vi "data_averaging.vi"(10 "Reset?":bool, 11 "New data":dbl[](array[numeric])) -> (3 "Output (averaged)":dbl[](array[numeric]))   [LabVIEW 2019]
uses:
  <vilib>/Analysis/baseanly.llb/Mean (DBL).vi
  Global Plantita Parameters.vi
  <vilib>/Analysis/NI_AALBase.lvlib
panel:
  out "Stored":dbl[](array[numeric])
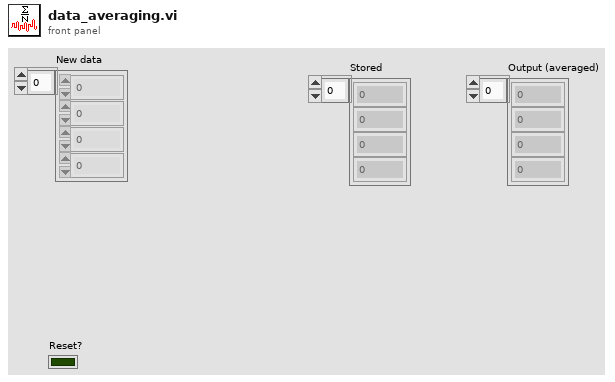
[diagram p1: front panel]
types:
  T1 = cluster{"height_ff (m)":dbl, "C_coag_stock (g/L)":dbl, "flocculation_time(min)":dbl, "clarification_time(min)":dbl, "data_interval (min)":dbl, "kpf":dbl, "kc":dbl, "q":dbl}
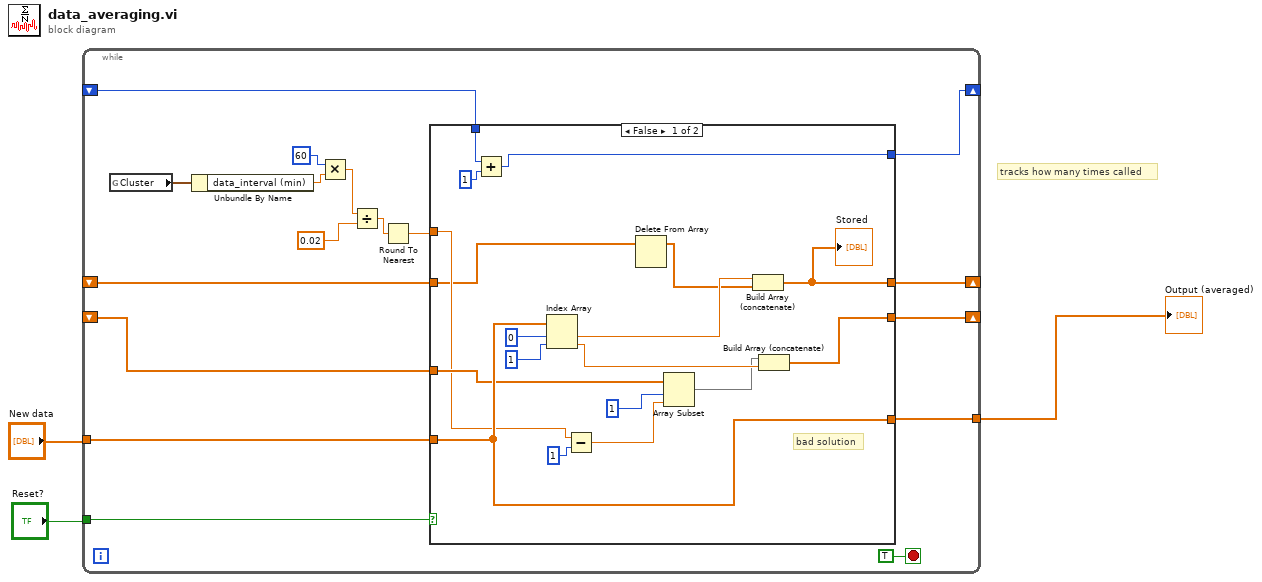
[diagram p0: block diagram]
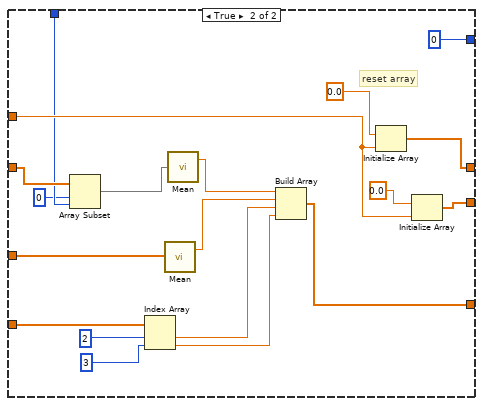
[diagram p2: hidden frame]
diagram:
  # "tracks how many times called"
  n1 = while {
    shift-right: [w15] -> _
    shift-left: _ -> [w16]
    tunnel: "Reset?" -> [w20]
    tunnel: "New data" -> [w19]
    tunnel: [w18] -> w2
    shift-right: [w13] -> _
    shift-left: _ -> [w14]
    shift-right: [w6] -> _
    shift-left: _ -> [w5]
    stop <- TRUE stop-if-true
    n2 = global read "Global Plantita Parameters.vi" "Cluster"() -> (w12:T1)
    n3 = Unbundle By Name(w12) -> ("data_interval (min)"=w11:dbl)
    n4 = Multiply(x=60, y=w11) -> (x*y=w9:dbl)
    n5 = Divide(x=w9, y=0.02) -> (x/y=w7:dbl)
    n6 = Round To Nearest(number=w7) -> (nearest integer value=w4:dbl)
    n7 = case shown="False" w20 {
      tunnel: w19 -> [w34 w54]
      tunnel: [w34 w55] -> w18
      tunnel: w16 -> [w24 w42]
      tunnel: w14 -> [w32 w47]
      tunnel: [w21 w51] -> w15
      tunnel: [w35 w50] -> w13
      tunnel: w4 -> [w29 w49]
      tunnel: [w25 0] -> w6
      tunnel: w5 -> [w26 w41]
      frame False {
        # "bad solution"
        n8 = Add(x=w26, y=1) -> (x+y=w25:i32)
        n9 = Index Array(array=w34, index #1=0, index #2=1) -> (element #1=w23:dbl, element #2=w36:dbl)
        n10 = Subtract(x=w29, y=1) -> (x-y=w28:dbl)
        n11 = Delete From Array(array=w24) -> (array with subset deleted=w22:dbl[])  [unwired: 2 in, 1 out]
        n12 = Array Subset(array=w32, index=1, length=w28) -> (w31:dbl[])
        n13 = Build Array (concatenate)(w23, w22) -> (w21:dbl[])
        "Stored" <- w21
        n14 = Build Array (concatenate)(w31, w36) -> (w35:dbl[])
      }
      frame True {
        # "reset array"
        n15 = Array Subset(array=w42, index=0, length=w41) -> (w40:dbl[])
        n16 = Index Array(array=w54, index #1=2, index #2=3) -> (element #1=w57:dbl, element #2=w44:dbl)
        n17 = call-poly <vilib>:"Mean.vi"("X"=w47) -> ("mean"=w46:dbl)  [unwired: 1 out]
        n18 = call-poly <vilib>:"Mean.vi"("X"=w40) -> ("mean"=w48:dbl)  [unwired: 1 out]
        n19 = Build Array(w48, w46, w57, w44) -> (w55:dbl[])
        n20 = Initialize Array(0.0, w49) -> (w51:dbl[])
        n21 = Initialize Array(0.0, w49) -> (w50:dbl[])
      }
    }
  }
  "Output (averaged)" <- w2
